vi "Field Update 4.3 to 5.0.vi"(8 "error in (no error)":errorcluster, 10 "Field Record":T2={"ixField"=0, "iSequenceOrder"=0, "sxFieldId"="", "sxSequenceId"="", "sDisplayName"="", "sValue"="", "sUnits"="", "nDataType"=enum."timestamp", "nNextItem"=enum."Reset", "fSystem"=FALSE, "fSystemValue"=FALSE, "fRequired"=FALSE, "fSetAtTest"=FALSE, "fTestField"=FALSE, "fDeleted"=FALSE, "fIndexed"=FALSE, "fFreeList"=FALSE} caption="Field Information", 11 "Connection Refnum":T1) -> (0 "error out":errorcluster, 3 "Connection Refnum":T1)   [LabVIEW 2011]
uses:
  Field Record.ctl
  Field DataTypes.ctl
  Field NextItem.ctl
  SI.LIB/ODBC/SQL Controls/Connection Refnum.ctl
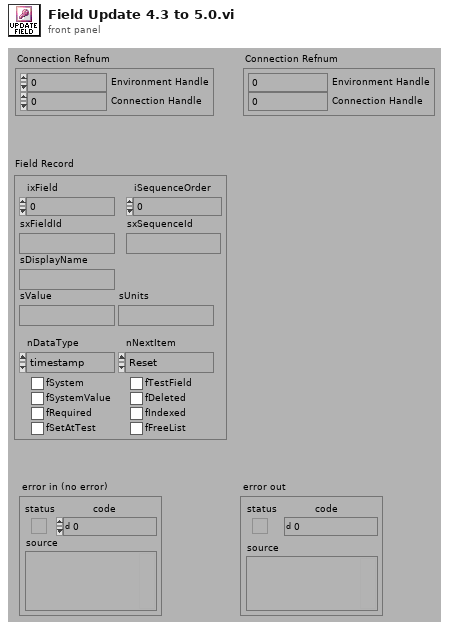
[diagram p1: front panel]
types:
  T1 = typedef "Connection Refnum.ctl" = cluster{"Environment Handle":i32, "Connection Handle":i32}
  T2 = typedef "Field Record.ctl" = cluster{"ixField":i32, "iSequenceOrder":i32, "sxFieldId":string, "sxSequenceId":string, "sDisplayName":string, "sValue":string, "sUnits":string, "nDataType":T3, "nNextItem":T4, "fSystem":bool, "fSystemValue":bool, "fRequired":bool, "fSetAtTest":bool, "fTestField":bool, "fDeleted":bool, "fIndexed":bool, "fFreeList":bool}
  T3 = typedef "Field DataTypes.ctl" = enum32{"text", "numeric", "list", "timestamp", "boolean"}
  T4 = typedef "Field NextItem.ctl" = enum32{"Reset", "Retain", "Auto-Increment"}
  T5 = typedef "Statement Refnum.ctl" = cluster{"Statement Handle":i32, "Parameter Number":u16}
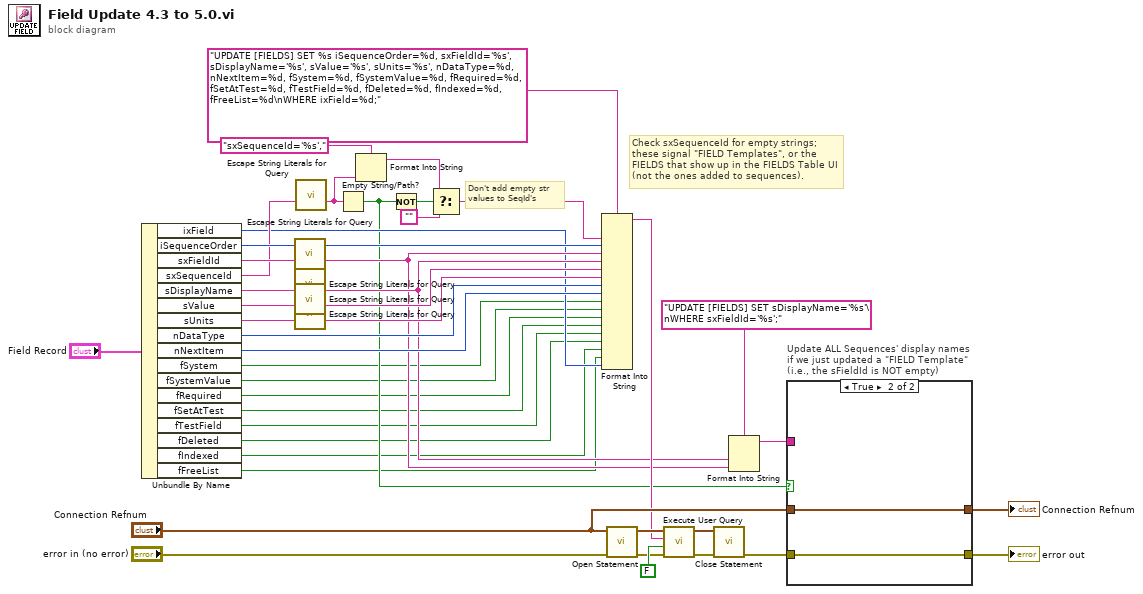
[diagram p0: block diagram]
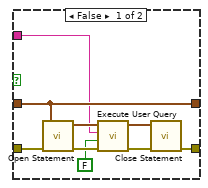
[diagram p2: hidden frame]
diagram:
  # "Don't add empty str\nvalues to SeqId's"
  # "Check sxSequenceId for empty strings;\nthese signal \"FIELD Templates\", or the\nFIELDS that show up in the FIELDS Table UI\n(not the ones added to sequences)."
  n1 = Unbundle By Name("Field Record") -> ("ixField"=w16:i32, "iSequenceOrder"=w30:i32, "sxFieldId"=w29:string, "sxSequenceId"=w28:string, "sDisplayName"=w27:string, "sValue"=w26:string, "sUnits"=w24:string, "nDataType"=w22:T3, "nNextItem"=w21:T4, "fSystem"=w9:bool, "fSystemValue"=w8:bool, "fRequired"=w7:bool, "fSetAtTest"=w6:bool, "fTestField"=w5:bool, "fDeleted"=w4:bool, "fIndexed"=w2:bool, "fFreeList"=w1:bool)
  n2 = call "Escape String Literals for Query.vi"("String"=w29) -> ("escaped String"=w17:string)  [unwired: 1 in, 13 out]
  n3 = call "Escape String Literals for Query.vi"("String"=w27) -> ("escaped String"=w18:string)  [unwired: 1 in, 13 out]
  n4 = call "Escape String Literals for Query.vi"("String"=w26) -> ("escaped String"=w25:string)  [unwired: 1 in, 13 out]
  n5 = call "Escape String Literals for Query.vi"("String"=w24) -> ("escaped String"=w23:string)  [unwired: 1 in, 13 out]
  n6 = call "Escape String Literals for Query.vi"("String"=w28) -> ("escaped String"=w14:string)  [unwired: 1 in, 13 out]
  n7 = Empty String/Path?(string/path=w14) -> (empty?=w13:bool)
  n8 = Format Into String(format string="sxSequenceId='%s'," ("User Query"), w14) -> (resulting string=w11:string)  [unwired: 2 in, 1 out]
  n9 = Not(x=w13) -> (.not. x?=w12:bool)
  n10 = Select(t=w11, s=w12, f="") -> (s? t:f=w3:string)
  n11 = Format Into String(format string="UPDATE [FIELDS] SET %s iSequenceOrder=%d, sxFieldId='%s', sDisplayName='%s', sValue='%s', sUnits='%s', nDataType=%d, nNextItem=%d, fSystem=%d, fSystemValue=%d, fRequired=%d, fSetAtTest=%d, fTestField=%d, fDeleted=%d, fIndexed=%d, fFreeList=%d\nWHERE ixField=%d;" ("User Query"), w3, w30, w17, w18, w25, w23, w22, w21, w9, w8, w7, w6, w5, w4, w2, w1, w16) -> (resulting string=w20:string)  [unwired: 2 in, 1 out]
  n12 = call "Open Statement.vi"("error in (no error)"="error in (no error)", "Connection Refnum"="Connection Refnum") -> ("error out"=w40:errorcluster, "Statement Refnum"=w39:T5)  [unwired: 4 out]
  n13 = call "Execute User Query.vi"("error in (no error)"=w40, "Return Data? (f)"=FALSE, "User Query"=w20, "Statement Refnum"=w39) -> ("error out"=w42:errorcluster, "Statement Refnum"=w41:T5)  [unwired: 2 out]
  n14 = call "Close Statement.vi"("error in (no error)"=w42, "Statement Refnum"=w41) -> ("error out"=w38:errorcluster)  [unwired: 5 out]
  n15 = Format Into String(format string="UPDATE [FIELDS] SET sDisplayName='%s'\nWHERE sxFieldId='%s';" ("User Query"), w18, w17) -> (resulting string=w19:string)  [unwired: 2 in, 1 out]
  n16 = case "Update ALL Sequences' display names\nif we just updated a \"FIELD Template\"\n(i.e., the sFieldId is NOT empty)" shown="True" w13 {
    tunnel: w38 -> [w47 w53]
    tunnel: "Connection Refnum" -> [w46 w54]
    tunnel: [w46 w54] -> w37
    tunnel: [w45 w53] -> w36
    tunnel: w19 -> [w44 _]
    frame False {
      n17 = call "Open Statement.vi"("error in (no error)"=w47, "Connection Refnum"=w46) -> ("error out"=w51:errorcluster, "Statement Refnum"=w52:T5)  [unwired: 4 out]
      n18 = call "Execute User Query.vi"("error in (no error)"=w51, "Return Data? (f)"=FALSE, "User Query"=w44, "Statement Refnum"=w52) -> ("error out"=w49:errorcluster, "Statement Refnum"=w50:T5)  [unwired: 2 out]
      n19 = call "Close Statement.vi"("error in (no error)"=w49, "Statement Refnum"=w50) -> ("error out"=w45:errorcluster)  [unwired: 5 out]
    }
    frame True {
    }
  }
  "error out" <- w36
  "Connection Refnum" <- w37
